vi "Explain Error Better.vi"(8 "User VI Ref":refnum<vi>, 9 "Error Cluster":errorcluster) -> ()   [LabVIEW 2020]
uses:
  <vilib>/Utility/error.llb/DialogTypeEnum.ctl
  <vilib>/Utility/error.llb/DialogType.ctl
  <vilib>/Utility/cursorutil.llb/Set Cursor (Icon Pict).vi
  <vilib>/Utility/inputDevices.llb/mouseAcquire.vi
  <vilib>/Utility/inputDevices.llb/closeKeyboard.vi
  <vilib>/Utility/inputDevices.llb/keyboardAcquire.vi
  <userlib>/_OpenG.lib/comparison/comparison.llb/I32 Changed__ogtk.vi
  <vilib>/Utility/inputDevices.llb/closeMouse.vi
  <vilib>/Platform/browser.llb/Open URL in Default Browser (string).vi
panel:
  in  "search google":bool
  out "Explanation":string
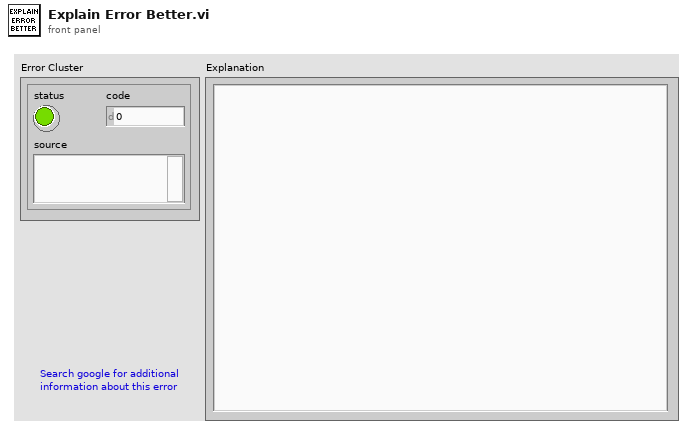
[diagram p1: front panel]
types:
  T1 = typedef "DialogTypeEnum.ctl" = enum16{"no dialog", "OK message", "continue or stop message", "auto error handling dialog", "OK message + warnings", "continue/stop + warnings"}
  T2 = typedef "DialogType.ctl" = u16
  T3 = cluster{"vi name":string, "start":i32, "end":i32}[]
  T4 = typedef "LVPoint32TypeDef.ctl" = cluster{"Horizontal":i32, "Vertical":i32}
  T5 = cluster{"button 1":bool, "button 2":bool, "button 3":bool, "button 4":bool}
  T6 = cluster{"vi name":string, "start":i32, "end":i32}
  T7 = enum16{"0", "1", "2", "3", "4", "5", "6", "7", "8", "9", "A", "B", "C", "D", "E", "F", "G", "H", "I", "J", "K", "L", "M", "N", "O", "P", "Q", "R", "S", "T", "U", "V", "W", "X", "Y", "Z", "F1", "F2", "F3", "F4", "F5", "F6", "F7", "F8", "F9", "F10", "F11", "F12", "F13", "F14", "F15", "ADD", "BACK", "BACKSLASH", "CAPITAL", "COMMA", "DECIMAL", "DELETE", "DIVIDE", "DOWN", "END", "EQUALS", "ESCAPE", "GRAVE (`)", "HOME", "INSERT", "LBRACKET", "LCONTROL", "LEFT", "L ALT", "LSHIFT", "LWIN", "MINUS", "MULTIPLY", "NEXT", "NUMLOCK", "NUMPAD_0", "NUMPAD_1", "NUMPAD_2", "NUMPAD_3", "NUMPAD_4", "NUMPAD_5", "NUMPAD_6", "NUMPAD_7", "NUMPAD_8", "NUMPAD_9", "PAUSE", "PERIOD", "PRIOR (PG UP)", "RBRACKET", "RCONTROL", "RETURN", "RIGHT", "R ALT", "RSHIFT", "RWIN", "SCROLL", "SEMICOLON", "SLASH", "SPACE", "SUBTRACT", "TAB", "UP", "ENTER (num pad)", "' (quote)"}[]
  T8 = cluster{"Shift":bool, "Ctrl":bool, "Alt":bool, "Cmd":bool, "Opt":bool}
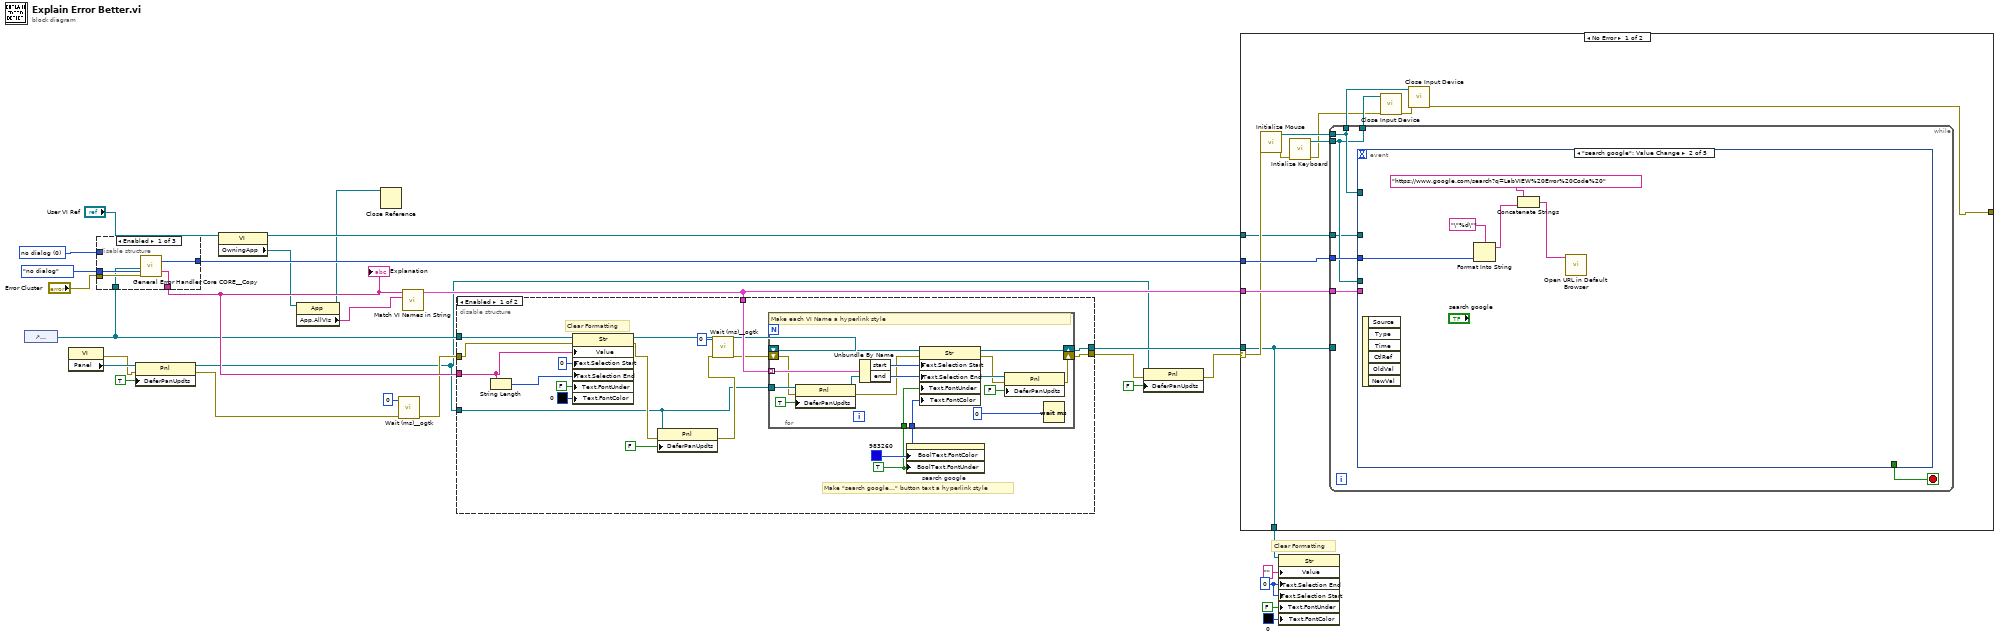
[diagram p0: block diagram]
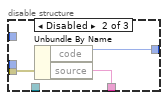
[diagram p3: hidden frame]
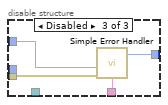
[diagram p4: hidden frame]
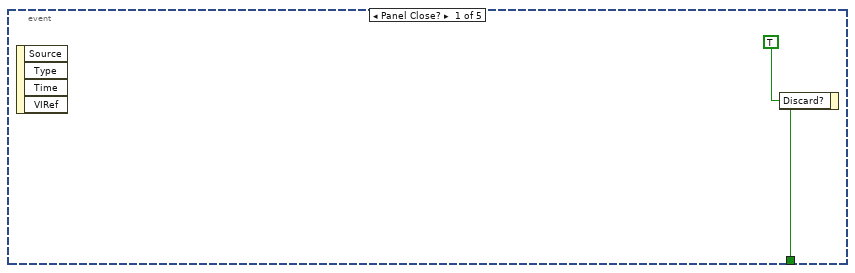
[diagram p5: hidden frame]
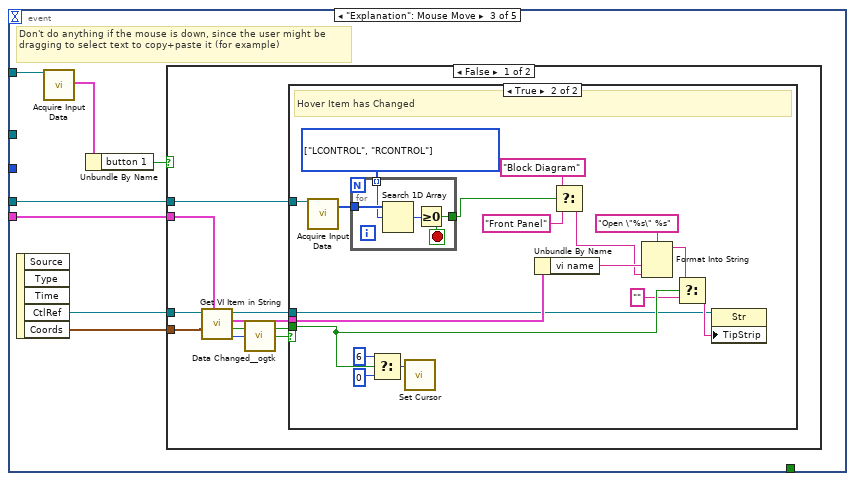
[diagram p6: hidden frame]
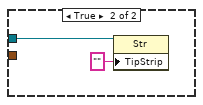
[diagram p8: hidden frame]
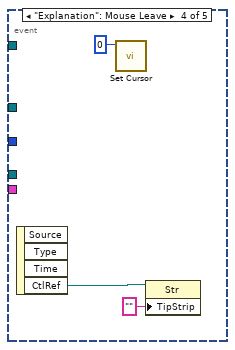
[diagram p9: hidden frame]
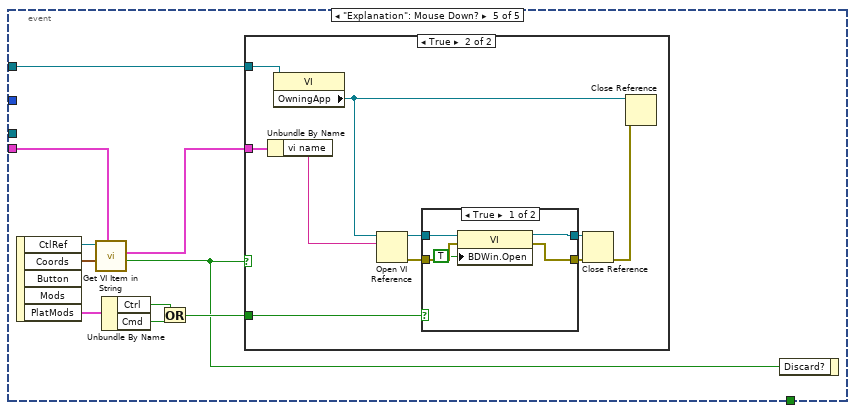
[diagram p10: hidden frame]
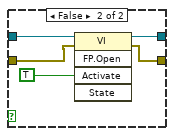
[diagram p12: hidden frame]
diagram:
  w16 = u32 0 ("Text.Selection:End")
  w23 = T2 0 items=["no dialog", "OK message", "continue or stop message", "OK message + warnings", "continue/stop + warnings"] ("type of dialog (OK msg:1)")
  # "Clear Formatting"
  n1 = control-ref of="Explanation"() -> (w20:refnum<vi>)
  n2 = property class="VI"() -> (error out=w12:errorcluster, "Panel"=w14:refnum<vi>)  [unwired: 2 in, 1 out]
  n3 = disable-structure shown="Enabled" {
    disable-tunnel: "Error Cluster" -> [w33 w36 w40]
    disable-tunnel: DialogTypeEnum."no dialog" ("type of dialog (OK msg:1)") -> [w32 _ _]
    disable-tunnel: [w31 w34 w39] -> w21
    disable-tunnel: [w30 w35 w38] -> w25
    disable-tunnel: w23 -> [_ _ w37]
    disable-tunnel: w20 -> [w29 _ _]
    frame Enabled {
      n4 = call <resource>:"General Error Handler Core CORE__Copy.vi"("String to Format (not a refnum)"=w29, "type of dialog (OK msg:1)"=w32, "error in (no error)"=w33) -> ("code out"=w30:i32, "message"=w31:string)  [unwired: 11 in, 4 out]
    }
    frame Disabled {
      n5 = Unbundle By Name(w36) -> ("code"=w35:i32, "source"=w34:string)
    }
    frame Disabled {
      n6 = call <vilib>:"Simple Error Handler.vi"("type of dialog (OK msg:1)"=w37, "error in (no error)"=w40) -> ("code out"=w38:i32, "message"=w39:string)  [unwired: 3 in, 3 out]
    }
  }
  "Explanation" <- w21
  n7 = property class="Pnl"(reference=w14, error in=w12, "DeferPanUpdts"=TRUE ("Defer Panel Updates")) -> (reference out=w5:refnum<vi>, error out=w7:errorcluster)
  n8 = property class="VI"(reference="User VI Ref") -> (reference out=w4:refnum<vi>, "OwningApp"=w3:refnum<vi>)  [unwired: 1 in, 1 out]
  n9 = property class="App"(reference=w3) -> (reference out=w1:refnum<vi>, "App.AllVIs"=w2:string[])  [unwired: 1 in, 1 out]
  n10 = Close Reference(reference=w1) -> ()  [unwired: 1 in, 1 out]
  n11 = call <userlib>:"Wait (ms)__ogtk.vi"("error in (no error)"=w7, "milliseconds to wait"=u32 0) -> ("error out"=w6:errorcluster)  [unwired: 8 in, 1 out]
  n12 = call <resource>:"Match VI Names in String.vi"("Application:All VIs In Memory"=w2, "string"=w21) -> ("vi names"=w28:T3)  [unwired: 9 in]
  n13 = disable-structure shown="Enabled" {
    disable-tunnel: w28 -> [w59 _]
    disable-tunnel: [w55 w76] -> w27
    disable-tunnel: [w52 _] -> w10
    disable-tunnel: w21 -> [w47 _]
    disable-tunnel: w20 -> [w51 w76]
    disable-tunnel: w6 -> [w50 _]
    disable-tunnel: w5 -> [w41 _]
    frame Enabled {
      w53 = TRUE ("Text.Font:Underline")
      w54 = u32 983260
      # "Make \"search google...\" button text a hyperlink style"
      # "Clear Formatting"
      n14 = String Length(string=w47) -> (length=w46:i32)
      n15 = property class="Str"(reference=w51, error in=w50, "Value"=w47, "Text.Selection Start"=u32 0 ("Text.Selection:Start"), "Text.Selection End"=w46, "Text.FontUnder"=FALSE ("Text.Font:Underline"), "Text.FontColor"=u32 0 ("Text.Font:Color")) -> (reference out=w58:refnum<vi>, error out=w43:errorcluster)
      n16 = property class="Pnl"(reference=w41, error in=w43, "DeferPanUpdts"=FALSE ("Defer Panel Updates")) -> (error out=w42:errorcluster)  [unwired: 1 out]
      n17 = call <userlib>:"Wait (ms)__ogtk.vi"("error in (no error)"=w42, "milliseconds to wait"=u32 0) -> ("error out"=w49:errorcluster)  [unwired: 8 in, 1 out]
      n18 = for {
        tunnel: w59 -> [w74] mode=indexing
        shift-right: [w71] -> w55
        shift-left: w58 -> [w75]
        tunnel: w54 -> [w70]
        tunnel: w53 -> [w69]
        shift-right: [w60] -> w52
        shift-left: w49 -> [w62]
        tunnel: w41 -> [w66]
        # "Make each VI Name a hyperlink style"
        n19 = property class="Pnl"(reference=w66, error in=w62, "DeferPanUpdts"=TRUE ("Defer Panel Updates")) -> (reference out=w64:refnum<vi>, error out=w63:errorcluster)
        n20 = Unbundle By Name(w74) -> ("start"=w73:i32, "end"=w72:i32)
        n21 = property class="Str"(reference=w75, error in=w63, "Text.Selection Start"=w73, "Text.Selection End"=w72, "Text.FontUnder"=w69, "Text.FontColor"=w70) -> (reference out=w71:refnum<vi>, error out=w61:errorcluster)
        n22 = property class="Pnl"(reference=w64, error in=w61, "DeferPanUpdts"=FALSE ("Defer Panel Updates")) -> (error out=w60:errorcluster)  [unwired: 1 out]
        n23 = Wait (ms)(milliseconds to wait=u32 0) -> ()  [unwired: 1 out]
      }
      n24 = property on="search google" class="Bool (strict)"("BoolText.FontColor"=w54, "BoolText.FontUnder"=w53) -> ()  [unwired: 2 in, 2 out]
    }
    frame Disabled {
    }
  }
  n25 = property class="Pnl"(reference=w5, error in=w10, "DeferPanUpdts"=FALSE ("Defer Panel Updates")) -> (error out=w9:errorcluster)  [unwired: 1 out]
  n26 = case shown="No Error" w9 {
    selector: w9 -> [w83 w176]
    tunnel: w28 -> [w89 _]
    tunnel: w27 -> [w77 w175]
    tunnel: w25 -> [w84 _]
    tunnel: [w78 w176] -> _
    tunnel: w4 -> [w79 _]
    tunnel: [w77 w175] -> w15
    frame No Error {
      n27 = call <vilib>:"Initialize Mouse.vi"("error in (no error)"=w83) -> ("error out"=w82:errorcluster, "device ID"=w88:refnum<k1>)  [unwired: 9 in]
      n28 = call <vilib>:"Intialize Keyboard.vi"("error in (no error)"=w82) -> ("error out"=w81:errorcluster, "device ID"=w86:refnum<k1>)  [unwired: 9 in]
      n29 = while {
        tunnel: w89 -> [w94]
        tunnel: w88 -> [w93]
        tunnel: [w93] -> w87
        tunnel: w77 -> [_]
        tunnel: w84 -> [w92]
        tunnel: w86 -> [w91]
        tunnel: [w91] -> w85
        tunnel: w79 -> [w90]
        stop <- w95 stop-if-true
        n30 = event shown="[1] \"search google\": Value Change" {
          selector: _ -> [_ _ _ _ _]
          dyn-events: _ -> [_ _ _ _ _]
          timeout: _ -> [_ _ _ _ _]
          tunnel: [w96 _ _ _ _] -> w95
          tunnel: w94 -> [_ _ w107 _ w153]
          tunnel: w93 -> [_ _ w105 _ _]
          tunnel: w92 -> [_ w101 _ _ _]
          tunnel: w91 -> [_ _ w102 _ _]
          tunnel: w90 -> [_ _ _ _ w146]
          event Panel Close? {
            w96 = TRUE ("Discard?")
            n31 = event-data() -> ()  [unwired: 1 in, 4 out]
            n32 = event-data("Discard?"=w96) -> ()  [unwired: 1 in, 1 out]
          }
          event "search google": Value Change {
            n33 = event-data() -> ()  [unwired: 1 in, 6 out]
            n34 = Format Into String(format string="\"%d\"", w101) -> (resulting string=w100:string)  [unwired: 2 in, 1 out]
            n35 = Concatenate Strings("https://www.google.com/search?q=LabVIEW%20Error%20Code%20" ("format string"), w100) -> (w98:string)
            n36 = call-poly <vilib>:"Open URL in Default Browser.vi"("URL"=w98) -> ()  [unwired: 5 in, 2 out]
          }
          event "Explanation": Mouse Move {
            # "Don't do anything if the mouse is down, since the user might be dragging to select text to copy+paste it (for example)"
            n37 = event-data() -> ("CtlRef"=w106:refnum<vi>, "Coords"=w108:T4)  [unwired: 1 in, 3 out]
            n38 = call-poly <vilib>:"Acquire Input Data.vi"("device ID"=w105) -> ("button info"=w104:T5)  [unwired: 15 in, 3 out]
            n39 = Unbundle By Name(w104) -> ("button 1"=w103:bool)
            n40 = case shown="False" w103 {
              tunnel: w108 -> [w117 _]
              tunnel: w107 -> [w116 _]
              tunnel: w106 -> [w112 w141]
              tunnel: w102 -> [w110 _]
              frame False {
                n41 = call <resource>:"Get VI Item in String.vi"("items"=w116, "Coords"=w117, "String in"=w112) -> ("item index"=w113:i32, "active item"=w114:bool, "item at coords"=w115:T6, "String out"=w109:refnum<vi>)  [unwired: 5 in]
                n42 = call-poly <userlib>:"Data Changed__ogtk.vi"("I32"=w113) -> ("Changed"=w111:bool)
                n43 = case shown="True" w111 {
                  tunnel: w115 -> [_ w131]
                  tunnel: w114 -> [_ w120]
                  tunnel: w110 -> [_ w128]
                  tunnel: w109 -> [_ w118]
                  frame False {
                  }
                  frame True {
                    w127 = T7 [enum."LCONTROL", enum."RCONTROL"] items=["0", "1", "2", "3", "4", "5", "6", "7", "8", "9", "A", "B", "C", "D", "E", "F", "G", "H", "I", "J", "K", "L", "M", "N", "O", "P", "Q", "R", "S", "T", "U", "V", "W", "X", "Y", "Z", "F1", "F2", "F3", "F4", "F5", "F6", "F7", "F8", "F9", "F10", "F11", "F12", "F13", "F14", "F15", "ADD", "BACK", "BACKSLASH", "CAPITAL", "COMMA", "DECIMAL", "DELETE", "DIVIDE", "DOWN", "END", "EQUALS", "ESCAPE", "GRAVE (`)", "HOME", "INSERT", "LBRACKET", "LCONTROL", "LEFT", "L ALT", "LSHIFT", "LWIN", "MINUS", "MULTIPLY", "NEXT", "NUMLOCK", "NUMPAD_0", "NUMPAD_1", "NUMPAD_2", "NUMPAD_3", "NUMPAD_4", "NUMPAD_5", "NUMPAD_6", "NUMPAD_7", "NUMPAD_8", "NUMPAD_9", "PAUSE", "PERIOD", "PRIOR (PG UP)", "RBRACKET", "RCONTROL", "RETURN", "RIGHT", "R ALT", "RSHIFT", "RWIN", "SCROLL", "SEMICOLON", "SLASH", "SPACE", "SUBTRACT", "TAB", "UP", "ENTER (num pad)", "' (quote)"] ("keys pressed")
                    # "Hover Item has Changed"
                    n44 = call-poly <vilib>:"Acquire Input Data.vi"("device ID"=w128) -> ("keys pressed"=w126:T7)  [unwired: 16 in, 2 out]
                    n45 = for {
                      tunnel: w127 -> [w138] mode=indexing
                      tunnel: w126 -> [w139]
                      tunnel: [w136] -> w125
                      stop <- w136 stop-if-true
                      n46 = Search 1D Array(1D array=w139, element=w138) -> (index of element=w137:i32)  [unwired: 1 in]
                      n47 = Greater Or Equal To 0?(x=w137) -> (x >= 0?=w136:bool)
                    }
                    n48 = Select(t=u16 6 ("icon"), s=w120, f=u16 0 ("icon")) -> (s? t:f=w133:u16)
                    n49 = call-poly <vilib>:"Set Cursor.vi"("icon"=w133) -> ()  [unwired: 9 in, 2 out]
                    n50 = Unbundle By Name(w131) -> ("vi name"=w130:string)
                    n51 = Select(t="Block Diagram" ("format string"), s=w125, f="Front Panel" ("format string")) -> (s? t:f=w122:string)
                    n52 = Format Into String(format string="Open \"%s\" %s", w130, w122) -> (resulting string=w121:string)  [unwired: 2 in, 1 out]
                    n53 = Select(t=w121, s=w120, f="" ("format string")) -> (s? t:f=w132:string)
                    n54 = property class="Str"(reference=w118, "TipStrip"=w132) -> ()  [unwired: 1 in, 2 out]
                  }
                }
              }
              frame True {
                n55 = property class="Str"(reference=w141, "TipStrip"="" ("Tip Strip")) -> ()  [unwired: 1 in, 2 out]
              }
            }
          }
          event "Explanation": Mouse Leave {
            n56 = event-data() -> ("CtlRef"=w142:refnum<vi>)  [unwired: 1 in, 3 out]
            n57 = call-poly <vilib>:"Set Cursor.vi"("icon"=u16 0) -> ()  [unwired: 9 in, 2 out]
            n58 = property class="Str"(reference=w142, "TipStrip"="" ("Tip Strip")) -> ()  [unwired: 1 in, 2 out]
          }
          event "Explanation": Mouse Down? {
            n59 = event-data() -> ("CtlRef"=w152:refnum<vi>, "Coords"=w154:T4, "PlatMods"=w151:T8)  [unwired: 1 in, 2 out]
            n60 = call <resource>:"Get VI Item in String.vi"("items"=w153, "Coords"=w154, "String in"=w152) -> ("active item"=w147:bool, "item at coords"=w145:T6)  [unwired: 5 in, 2 out]
            n61 = Unbundle By Name(w151) -> ("Ctrl"=w149:bool, "Cmd"=w150:bool)
            n62 = Or(x=w149, y=w150) -> (x .or. y?=w148:bool)
            n63 = case shown="True" w147 {
              tunnel: w148 -> [_ w160]
              tunnel: w146 -> [_ w157]
              tunnel: w145 -> [_ w159]
              frame False {
              }
              frame True {
                n64 = Unbundle By Name(w159) -> ("vi name"=w158:string)
                n65 = property class="VI"(reference=w157) -> ("OwningApp"=w156:refnum<vi>)  [unwired: 1 in, 2 out]
                n66 = Open VI Reference(application reference (local)=w156, vi path=w158) -> (vi reference=w164:refnum<vi>, error out=w163:errorcluster)  [unwired: 4 in]
                n67 = case shown="True" w160 {
                  tunnel: w164 -> [w169 w174]
                  tunnel: w163 -> [w168 w172]
                  tunnel: [w166 w171] -> w162
                  tunnel: [w165 w170] -> w161
                  frame True {
                    n68 = property class="VI"(reference=w169, error in=w168, "BDWin.Open"=TRUE ("Block Diagram Window:Open")) -> (reference out=w165:refnum<vi>, error out=w166:errorcluster)
                  }
                  frame False {
                    n69 = invoke class="VI" method="FP.Open"(reference=w174, error in=w172, "Activate"=TRUE ("Activate?")) -> (reference out=w170:refnum<vi>, error out=w171:errorcluster)  [unwired: 2 in, 3 out]
                  }
                }
                n70 = Close Reference(reference=w161, error in (no error)=w162) -> (error out=w155:errorcluster)
                n71 = Close Reference(reference=w156, error in (no error)=w155) -> ()  [unwired: 1 out]
              }
            }
            n72 = event-data("Discard?"=w147) -> ()  [unwired: 1 in, 1 out]
          }
        }
      }
      n73 = call-poly <vilib>:"Close Input Device.vi"("error in (no error)"=w81, "device ID"=w85) -> ("error out"=w80:errorcluster)  [unwired: 8 in]
      n74 = call-poly <vilib>:"Close Input Device.vi"("error in (no error)"=w80, "device ID"=w87) -> ("error out"=w78:errorcluster)  [unwired: 8 in]
    }
    frame Error {
    }
  }
  n75 = property class="Str"(reference=w15, "Value"="", "Text.Selection End"=w16, "Text.Selection Start"=w16, "Text.FontUnder"=FALSE ("Text.Font:Underline"), "Text.FontColor"=u32 0 ("Text.Font:Color")) -> ()  [unwired: 1 in, 2 out]
